vi "DllFxpIntAccumulator_BoolArray.vi"(6 "enable":bool, 8 "cinNbin":bool, 9 "isSub":bool, 10 "load":bool, 11 "x":bool[](array[boolean])=[FALSE, FALSE, FALSE, FALSE, FALSE, FALSE, FALSE, FALSE, FALSE, FALSE, FALSE, FALSE, FALSE, FALSE, FALSE, FALSE]) -> (2 "coutNbout":bool, 3 "sum":bool[](array[boolean]))   [LabVIEW 2017]
uses:
  <vilib>/rvi/FXPMathLib/basic elements/FxpIntAccumulator/subVIs/nifxpmath_IntAccumulator_SimConfig.ctl
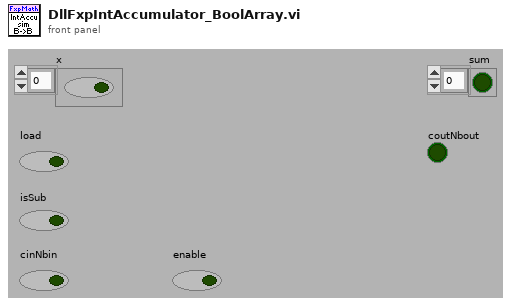
[diagram p1: front panel]
types:
  T1 = typedef "nifxpmath_IntAccumulator_SimConfig.ctl" = cluster{"kWordLengthIn":u16, "kWordLengthOut":u16, "kPrescaling":u16, "kNumOfCh":u16, "kIsSigned":bool, "kIsRegOut":bool}
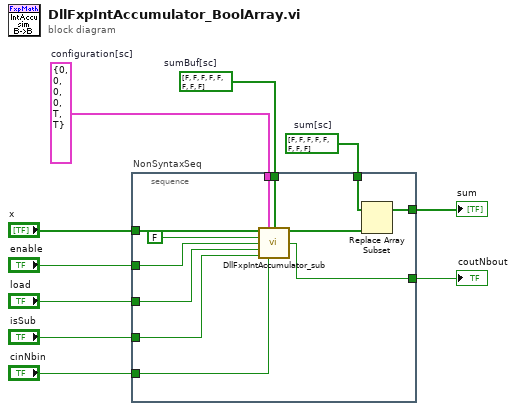
[diagram p0: block diagram]
diagram:
  w4 = bool[] [FALSE, FALSE, FALSE, FALSE, FALSE, FALSE, FALSE, FALSE]  # sum[sc]
  w2 = bool[] [FALSE, FALSE, FALSE, FALSE, FALSE, FALSE, FALSE, FALSE]  # sumBuf[sc]
  w8 = T1 {"kWordLengthIn"=0, "kWordLengthOut"=0, "kPrescaling"=0, "kNumOfCh"=0, "kIsSigned"=TRUE, "kIsRegOut"=TRUE}  # configuration[sc]
  n1 = stacked-sequence "NonSyntaxSeq" {
    tunnel: [w12] -> w9
    tunnel: "load" -> [w15]
    tunnel: "enable" -> [w16]
    tunnel: "x" -> [w18]
    tunnel: w8 -> [w20]
    tunnel: w4 -> [w22]
    tunnel: "cinNbin" -> [w13]
    tunnel: "isSub" -> [w14]
    tunnel: [w21] -> w3
    tunnel: w2 -> [w19]
    frame #0 {
      n2 = call <vilib>:"DllFxpIntAccumulator_sub.vi"("x"=w18, "configuration[sc]"=w20, "sumBuf[sc]"=w19, "xov"=FALSE, "enable"=w16, "load"=w15, "isSub"=w14, "cinNbin"=w13) -> ("s"=w11:bool[], "coutNbout"=w12:bool)  [unwired: 1 in, 5 out]
      n3 = Replace Array Subset(array=w22, new element=w11) -> (w21:bool[])  [unwired: 1 in]
    }
  }
  "coutNbout" <- w9
  "sum" <- w3
